vi "Read Start Time.vi"(8 "error in (no error)":errorcluster, 11 "AcquistionObject in":refnum<class "AcquistionObject.lvclass">) -> (0 "error out":errorcluster, 2 "Start Time":timestamp, 3 "AcquistionObject out":refnum<class "AcquistionObject.lvclass">)   [LabVIEW 2010, in "AcquistionObject.lvclass"]
uses:
  AcquistionObject.lvclass
  AcquistionObject.lvclass/AcquistionObject.ctl
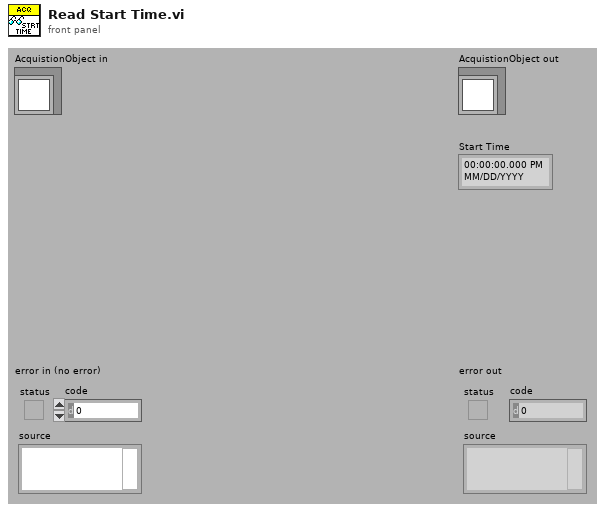
[diagram p1: front panel]
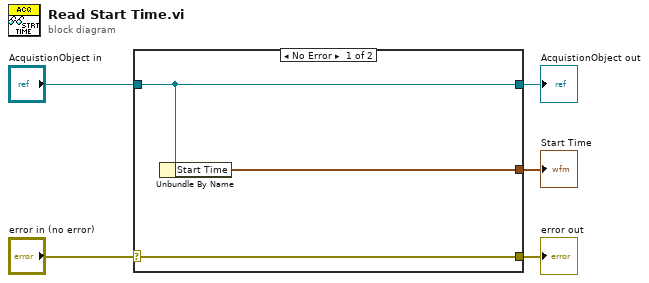
[diagram p0: block diagram]
diagram:
  n1 = case shown="No Error" "error in (no error)" {
    selector: "error in (no error)" -> [w8 w9]
    tunnel: [w8 w9] -> w4
    tunnel: [w7 w10] -> w2
    tunnel: "AcquistionObject in" -> [w7 w10]
    tunnel: [w6 _] -> w1
    frame No Error {
      n2 = Unbundle By Name(w7) -> ("Start Time"=w6:timestamp)
    }
    frame Error {
    }
  }
  "error out" <- w4
  "AcquistionObject out" <- w2
  "Start Time" <- w1
